vi "SlowNearWaypoint.vi"(8 "Yrobot":dbl, 9 "Xrobot":dbl, 10 "Ywaypoint":dbl, 11 "Xwaypoiny":dbl) -> (3 "SpeedDecrease":i32)   [LabVIEW 2012]
doc: "This VI checks to see if the robots curretn position is close to the next waypoint. If it is, it sets a boolean flag to allow a case statement to slow down robot"
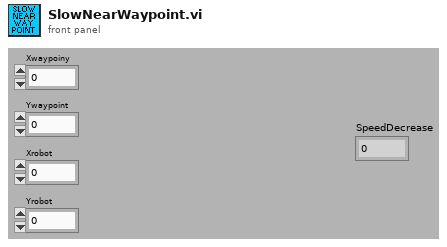
[diagram p1: front panel]
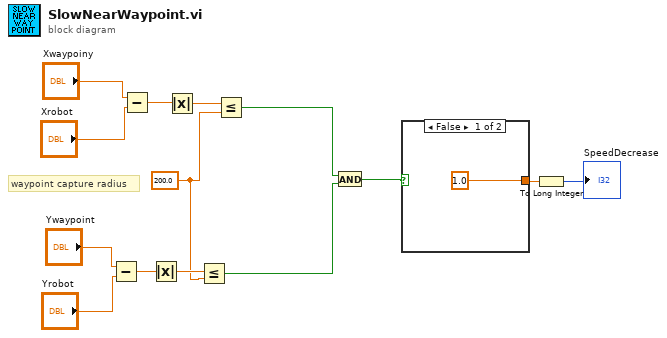
[diagram p0: block diagram]
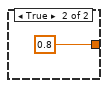
[diagram p2: hidden frame]
diagram:
  w6 = 200.0 ("y")
  # "waypoint capture radius"
  n1 = Subtract(x="Ywaypoint", y="Yrobot") -> (x-y=w9:dbl)
  n2 = Subtract(x="Xwaypoiny", y="Xrobot") -> (x-y=w10:dbl)
  n3 = Absolute Value(x=w9) -> (abs(x)=w8:dbl)
  n4 = Absolute Value(x=w10) -> (abs(x)=w7:dbl)
  n5 = Less Or Equal?(x=w8, y=w6) -> (x <= y?=w4:bool)
  n6 = Less Or Equal?(x=w7, y=w6) -> (x <= y?=w5:bool)
  n7 = And(x=w5, y=w4) -> (x .and. y?=w3:bool)
  n8 = case shown="False" w3 {
    tunnel: [1.0 0.8] -> w2
    frame False {
    }
    frame True {
    }
  }
  n9 = To Long Integer(number=w2) -> (32bit integer=→"SpeedDecrease":i32)
